vi "_readValue.vi"(8 "error in (no error)":errorcluster, 10 "Token Type":T1=enum."Other", 11 "JSONParser in":refnum<class "tJSONParser.lvclass">) -> (0 "error out":errorcluster, 2 "tBSONElement Out":refnum<class "tBSONElement.lvclass">, 3 "JSONParser out":refnum<class "tJSONParser.lvclass">)   [LabVIEW 2013, in "JSON.lvlib" / "tJSONParser.lvclass"]
doc: "Reads the value in a string : value pair and returns it in a tBSONElement object for storage in the tBSONDocument object."
uses:
  tJSONParser.lvclass
  BSON/tBSONElement/tBSONElement.lvclass
  _tokenType.ctl
  BSON/BSONElements/tBSONDocumentElement/tBSONDocumentElement.lvclass
  BSON/BSONElements/tBSONString/tBSONString.lvclass
  _error.ctl
  BSON/BSONElements/tBSONDocumentElement/setValue.vi
  BSON/BSONElements/tBSONString/setValue.vi
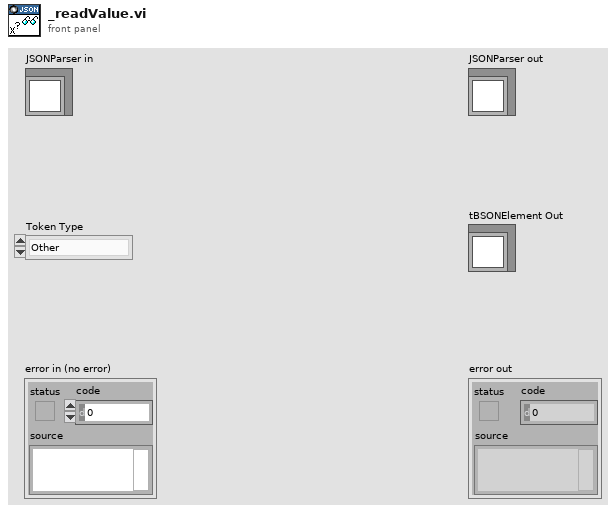
[diagram p1: front panel]
types:
  T1 = typedef "JSON.lvlib/tJSONParser.lvclass/_tokenType.ctl" = enum16{"Object Begin", "Object End", "Array Begin", "Array End", "String Delimeter", "Forward Slash", "Number", "Boolean", "Null", "Object Or Array Separator", "Pair Separator", "End Of File", "Asterisk", "Backward Slash", "Other"}
  T2 = typedef "JSON.lvlib/tJSONParser.lvclass/_error.ctl" = enum16{"Missing Object Open", "Missing Pair Separator", "Missing Object End Or Separator", "Missing Pair String", "Unexpected Token", "Missing Array End Or Separator", "Invalid Escape Sequence", "Unexpected End Of File", "Invalid Unicode", "Unexpected End Of Line", "Invalid Numerical Constant"}
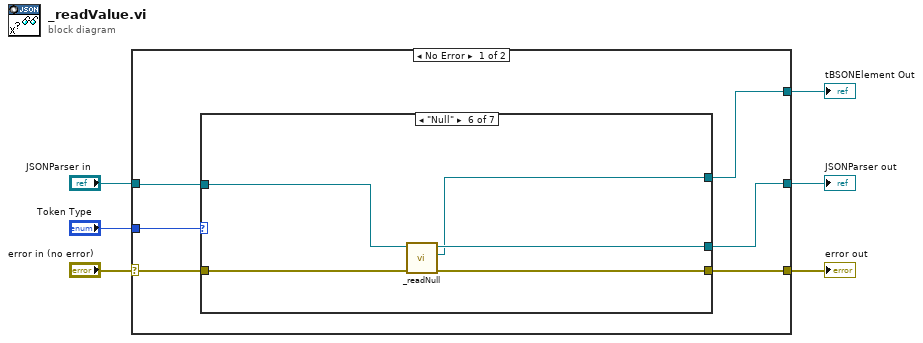
[diagram p0: block diagram]
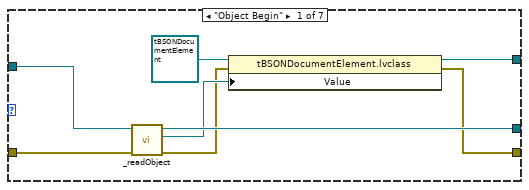
[diagram p2: hidden frame]
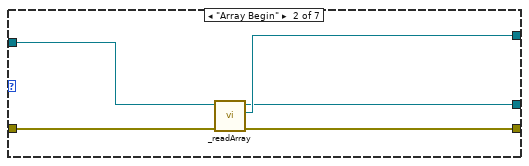
[diagram p3: hidden frame]
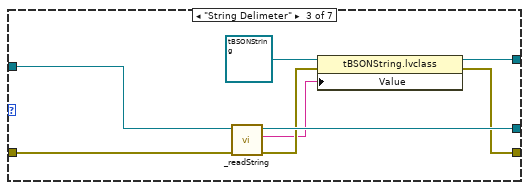
[diagram p4: hidden frame]
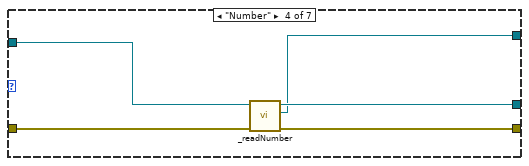
[diagram p5: hidden frame]
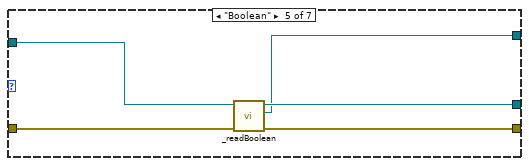
[diagram p6: hidden frame]
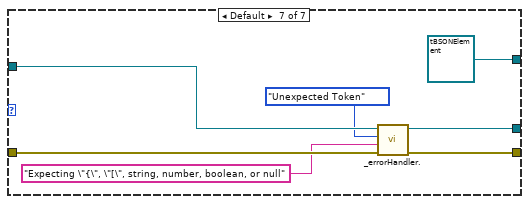
[diagram p7: hidden frame]
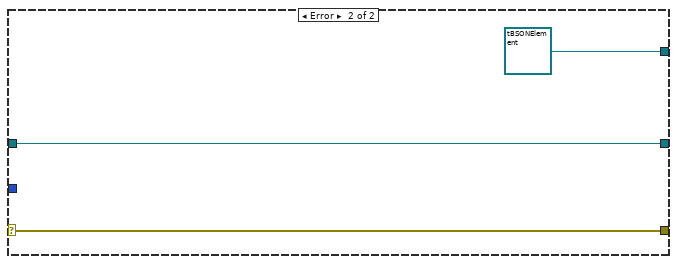
[diagram p8: hidden frame]
diagram:
  n1 = case shown="No Error" "error in (no error)" {
    selector: "error in (no error)" -> [w7 w58]
    tunnel: [w12 w58] -> w5
    tunnel: [w11 w57] -> w3
    tunnel: "JSONParser in" -> [w8 w57]
    tunnel: [w10 refnum<class "tBSONElement.lvclass"> refnum ("tBSONElement Out")] -> w2
    tunnel: "Token Type" -> [w9 _]
    frame No Error {
      n2 = case shown="\"Null\"" w9 {
        tunnel: w7 -> [w20 w22 w33 w36 w41 w46 w55]
        tunnel: [w14 w21 w27 w35 w40 w45 w54] -> w12
        tunnel: w8 -> [w19 w24 w32 w37 w43 w48 w53]
        tunnel: [w18 w23 w31 w38 w42 w47 w52] -> w11
        tunnel: [w13 w25 w29 w34 w39 w44 refnum<class "tBSONElement.lvclass"> refnum ("lvMongoDriver.lvlib:BSON.lvlib:tBSONElement.lvclass")] -> w10
        frame "Object Begin" {
          n3 = call "_readObject.vi"("error in (no error)"=w20, "JSONParser in"=w19) -> ("error out"=w15:errorcluster, "tBSONDocument out"=w16:refnum<class "tBSONDocument.lvclass">, "JSONParser out"=w18:refnum<class "tJSONParser.lvclass">)  [unwired: 7 in]
          n4 = property class="tBSONDocumentElement.lvclass"(reference=refnum<class "tBSONDocumentElement.lvclass"> refnum, error in=w15, "Value"=w16) -> (reference out=w13:refnum<class "tBSONDocumentElement.lvclass">, error out=w14:errorcluster)
        }
        frame "Array Begin" {
          n5 = call "_readArray.vi"("error in (no error)"=w22, "JSONParser in"=w24) -> ("error out"=w21:errorcluster, "tBSONArray Out"=w25:refnum<class "tBSONArray.lvclass">, "JSONParser out"=w23:refnum<class "tJSONParser.lvclass">)  [unwired: 7 in]
        }
        frame "String Delimeter" {
          n6 = call "_readString.vi"("error in (no error)"=w33, "JSONParser in"=w32) -> ("error out"=w28:errorcluster, "String"=w26:string, "JSONParser out"=w31:refnum<class "tJSONParser.lvclass">)  [unwired: 7 in]
          n7 = property class="tBSONString.lvclass"(reference=refnum<class "tBSONString.lvclass"> refnum ("lvMongoDriver.lvlib:BSON.lvlib:tBSONString.lvclass"), error in=w28, "Value"=w26) -> (reference out=w29:refnum<class "tBSONString.lvclass">, error out=w27:errorcluster)
        }
        frame "Number" {
          n8 = call "_readNumber.vi"("error in (no error)"=w36, "tJSONParser in"=w37) -> ("error out"=w35:errorcluster, "tBSONElement Out"=w34:refnum<class "tBSONElement.lvclass">, "tJSONParser out"=w38:refnum<class "tJSONParser.lvclass">)  [unwired: 7 in]
        }
        frame "Boolean" {
          n9 = call "_readBoolean.vi"("error in (no error)"=w41, "tJSONParser in"=w43) -> ("error out"=w40:errorcluster, "tBSONBoolean out"=w39:refnum<class "tBSONBoolean.lvclass">, "tJSONParser out"=w42:refnum<class "tJSONParser.lvclass">)  [unwired: 7 in]
        }
        frame "Null" {
          n10 = call "_readNull.vi"("error in (no error)"=w46, "tJSONParser in"=w48) -> ("error out"=w45:errorcluster, "tBSONNull out"=w44:refnum<class "tBSONNull.lvclass">, "tJSONParser out"=w47:refnum<class "tJSONParser.lvclass">)  [unwired: 7 in]
        }
        frame Default {
          n11 = call "_errorHandler..vi"("error in (no error)"=w55, "Additional Text"="Expecting \"{\", \"[\", string, number, boolean, or null", "Error Type"=_error."Unexpected Token", "JSON Parser In"=w53) -> ("error out"=w54:errorcluster, "JSON Parser Out"=w52:refnum<class "tJSONParser.lvclass">)  [unwired: 6 in]
        }
      }
    }
    frame Error {
    }
  }
  "error out" <- w5
  "JSONParser out" <- w3
  "tBSONElement Out" <- w2
